vi "Parse.vi"(8 "Error In":errorcluster, 11 "object in":refnum<class "2024_10.lvclass">) -> (0 "Error Out":errorcluster, 3 "object out":refnum<class "2024_10.lvclass">)   [LabVIEW 2023, in "2024_10.lvclass"]
uses:
  2024_10.lvclass
  2024_10.lvclass/2024_10.ctl
  <userlib>/_OpenG.lib/string/string.llb/openg_string.lvlib
panel:
  out "Array":u8[][](array[numeric])
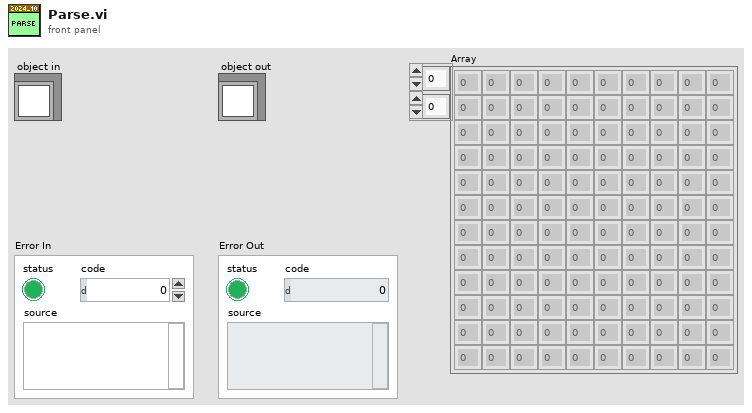
[diagram p1: front panel]
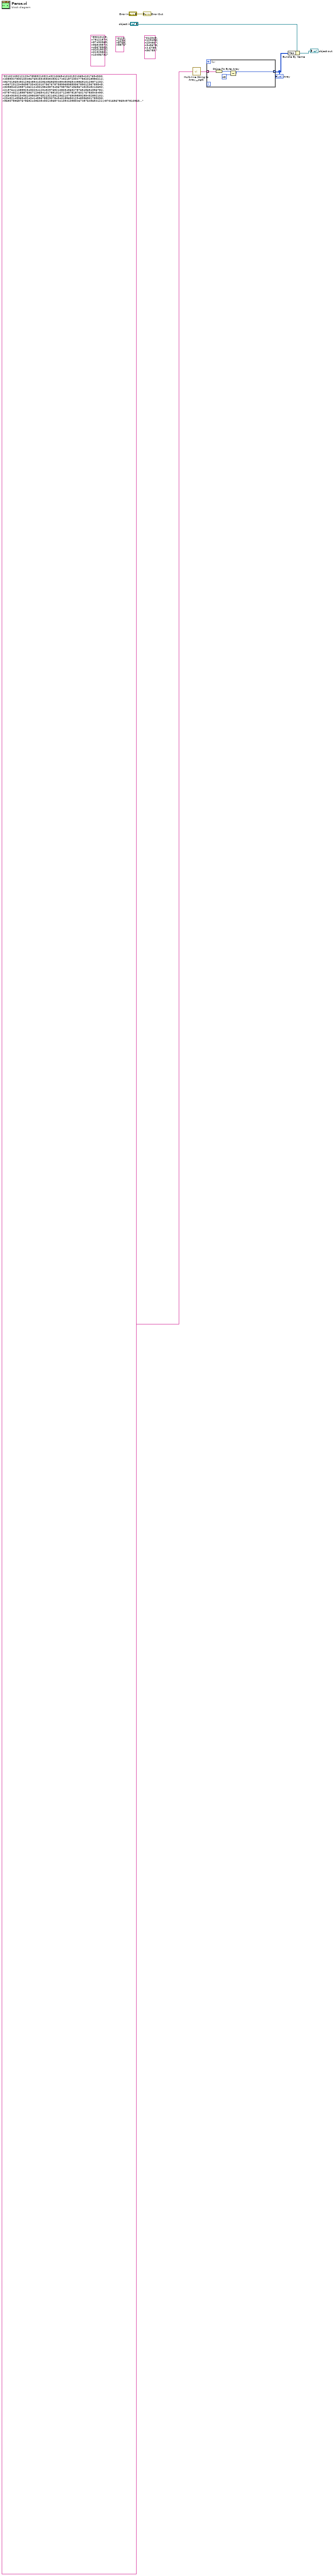
[diagram p0: block diagram]
diagram:
  (unwired) "012345\n123456\n234567\n345678\n4.6789\n56789."
  (unwired) "89010123\n78121874\n87430965\n96549874\n45678903\n32019012\n01329801\n10456732"
  (unwired) "0123\n1234\n8765\n9876"
  n1 = call <userlib>:"Multi-line String to Array__ogtk.vi"("string"="321021092121234789832103214321006541010132106541017654300\n438934783010345676543345305453217432187233477832018980211\n567015654501296489410256456569348945096544986910129871232\n456723123456987334320107567678758996898555678901236789543\n309854010987106212430198438734367987567456967432545210692\n219764110899234302341234329765210803456327876545694356781\n078743211898765671296541017891010712987818760176783543490\n165430302345610980387652132169125621076909859285432892101\n234321459654324341455678923078434018565012348396501783030\n965078968767865210564543014568742109410983467487645654121\n87016567865497810963..." ("PuzzleInput")) -> ("lines"=w3:string[])
  n2 = for {
    tunnel: w3 -> [w10] mode=indexing
    tunnel: [w7] -> w2 mode=indexing
    n3 = String To Byte Array(string=w10) -> (unsigned byte array=w9:u8[])
    n4 = Subtract(x=w9, y=u8 48) -> (x-y=w7:u8[])
  }
  "Array" <- w2
  n5 = Bundle By Name(cluster="object in", "Map"=w2) -> (→"object out":refnum<class "2024_10.lvclass">)
  "Error Out" <- "Error In"
